vi "Write Pointer.vi"(8 "error in (no error)":errorcluster, 10 "Pointer":i64, 11 "Pointer Base in":refnum<class "Pointer Base.lvclass">) -> (0 "error out":errorcluster, 3 "Pointer Base out":refnum<class "Pointer Base.lvclass">)   [LabVIEW 2020, in "PV Access.lvlib" / "Pointer Base.lvclass"]
uses:
  Pointer Base.lvclass
  Pointer Base.lvclass/Pointer Base.ctl
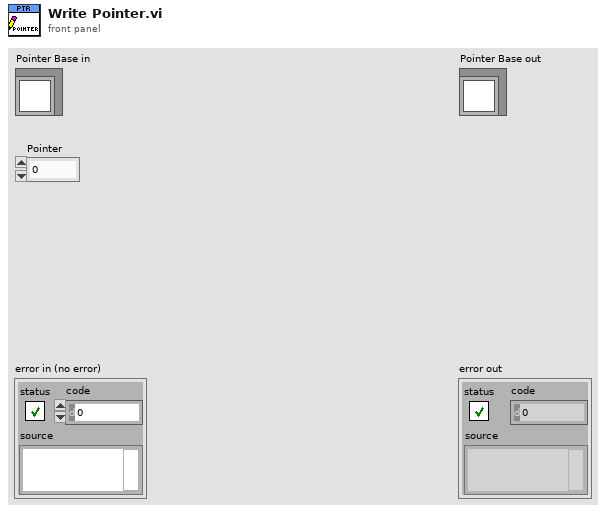
[diagram p1: front panel]
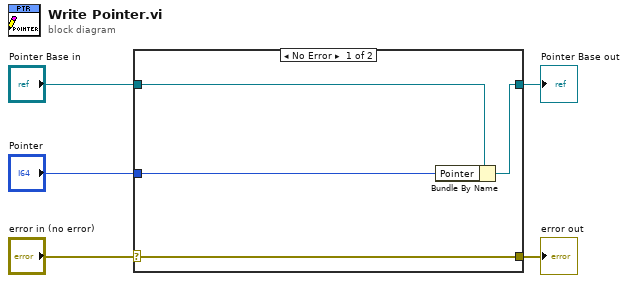
[diagram p0: block diagram]
diagram:
  n1 = case shown="No Error" "error in (no error)" {
    selector: "error in (no error)" -> [w9 w10]
    tunnel: [w9 w10] -> w4
    tunnel: [w7 w11] -> w2
    tunnel: "Pointer Base in" -> [w8 w11]
    tunnel: "Pointer" -> [w6 _]
    frame No Error {
      n2 = Bundle By Name(cluster=w8, "Pointer"=w6) -> (w7:refnum<class "Pointer Base.lvclass">)
    }
    frame Error {
    }
  }
  "error out" <- w4
  "Pointer Base out" <- w2
